vi "Messages GUI.vi"(11 "Messages":string) -> ()   [LabVIEW 2013]
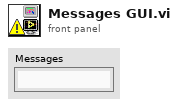
[diagram p1: front panel]
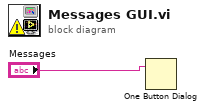
[diagram p0: block diagram]
diagram:
  n1 = One Button Dialog(message="Messages") -> ()  [unwired: 1 in, 1 out]
